vi "SVFA Get Spectrum Subset (1 Ch).vi"(0 "spectrum":cluster{"x0":dbl, "dx":dbl, "magnitude":dbl[]} {"magnitude" format="%.2f"; "dx" format="%.2f"; "x0" format="%.2f"}, 2 "range":cluster{"start":dbl, "stop":dbl}={"start"=-1.0, "stop"=-1.0} {"stop" format="%.2f"; "start" format="%.2f"}, 4 "spectrum info":T1={"channel name"="", "description"="", "x-axis units"=0, "spectral info"={"spectrum type"=enum."Power [Magnitude^2]", "linear/dB"=enum."linear", "window"=0, "window size"=0, "FFT size"=0}, "engineering units"=0, "custom label"="", "dB reference [EU]"=0.0, "peak units"=enum."rms", "weighting filter"=0, "spectral density?"=FALSE, "unit label"="", "spectrum skewed?"=FALSE, "complimentary spectrum units"=enum."none"} {"x-axis units" items=["Frequency-CB (Hz)"=0, "Frequency-CB (Hz)"=1, "Frequency-CPB (Hz)"=1248, "Frequency-Arbitrary (Hz)"=2357, "Quefrency (s)"=2, "Revolutions (rev)"=3, "Order"=4, "Speed (RPM)"=11, "Speed (rad/s)"=21, "Index"=65535]; "weighting filter" items=["Linear", "A-weighting", "B-weighting", "C-weighting", "ITU-R 468-4", "Dolby", "CCITT", "C-message", "Wb", "Wc", "Wd", "We", "Wf", "Wh", "Wj", "Wk", "Wm", "AES17 20 kHz lowpass", "AES17 40 kHz lowpass", "AES17 20 kHz highpass", "AES17 40 kHz highpass"]; "dB reference [EU]" format="%.2f"; "engineering units" items=["custom..."=0, "V"=1, "A"=21, "C"=30, "pC"=31, "s"=32, "-"=29, "Pa"=2, "N"=20, "g"=3, "m/s^2"=4, "m/s"=5, "m"=6, "mm/s"=12, "mm"=13, "micron/s"=14, "micron"=15, "in/s^2"=7, "in/s"=8, "in"=9, "mil/s"=10, "mil"=11, "rad/s^2"=16, "rad/s"=17, "rad"=18, "deg/s^2"=26, "deg/s"=27, "deg"=28, "RPM"=22, "cycle/s^2"=23, "Hz"=24, "cycle"=25, "strain"=19]; "spectral info"."window" items=["None "=0, "Hanning"=1, "Hamming"=2, "Blackman-Harris"=3, "Exact Blackman"=4, "Blackman"=5, "Flat Top"=6, "4 Term B-Harris "=7, "7 Term B-Harris"=8, "Low Sidelobe"=9, "Force - Exponential"=10, "Gaussian"=62]}, 5 "error in (no error)":errorcluster) -> (14 "spectrum subset":cluster{"x0":dbl, "dx":dbl, "magnitude":dbl[]} {"magnitude" format="%.2f"; "dx" format="%.2f"; "x0" format="%.2f"}, 15 "unit label":string, 16 "actual range":cluster{"start":dbl, "stop":dbl}={"start"=-1.0, "stop"=-1.0} {"stop" format="%.2f"; "start" format="%.2f"}, 17 "range label":string, 18 "dup spectrum info":T1={"channel name"="", "description"="", "x-axis units"=0, "spectral info"={"spectrum type"=enum."Power [Magnitude^2]", "linear/dB"=enum."linear", "window"=0, "window size"=0, "FFT size"=0}, "engineering units"=0, "custom label"="", "dB reference [EU]"=0.0, "peak units"=enum."rms", "weighting filter"=0, "spectral density?"=FALSE, "unit label"="", "spectrum skewed?"=FALSE, "complimentary spectrum units"=enum."none"} {"x-axis units" items=["Frequency-CB (Hz)"=0, "Frequency-CB (Hz)"=1, "Frequency-CPB (Hz)"=1248, "Frequency-Arbitrary (Hz)"=2357, "Quefrency (s)"=2, "Revolutions (rev)"=3, "Order"=4, "Speed (RPM)"=11, "Speed (rad/s)"=21, "Index"=65535]; "weighting filter" items=["Linear", "A-weighting", "B-weighting", "C-weighting", "ITU-R 468-4", "Dolby", "CCITT", "C-message", "Wb", "Wc", "Wd", "We", "Wf", "Wh", "Wj", "Wk", "Wm", "AES17 20 kHz lowpass", "AES17 40 kHz lowpass", "AES17 20 kHz highpass", "AES17 40 kHz highpass"]; "dB reference [EU]" format="%.2f"; "engineering units" items=["custom..."=0, "V"=1, "A"=21, "C"=30, "pC"=31, "s"=32, "-"=29, "Pa"=2, "N"=20, "g"=3, "m/s^2"=4, "m/s"=5, "m"=6, "mm/s"=12, "mm"=13, "micron/s"=14, "micron"=15, "in/s^2"=7, "in/s"=8, "in"=9, "mil/s"=10, "mil"=11, "rad/s^2"=16, "rad/s"=17, "rad"=18, "deg/s^2"=26, "deg/s"=27, "deg"=28, "RPM"=22, "cycle/s^2"=23, "Hz"=24, "cycle"=25, "strain"=19]; "spectral info"."window" items=["None "=0, "Hanning"=1, "Hamming"=2, "Blackman-Harris"=3, "Exact Blackman"=4, "Blackman"=5, "Flat Top"=6, "4 Term B-Harris "=7, "7 Term B-Harris"=8, "Low Sidelobe"=9, "Force - Exponential"=10, "Gaussian"=62]}, 19 "error out":errorcluster)   [LabVIEW 2017]
doc: "Extracts the subset of the spectrum specified by <B>range</B>. <B>x0</B> is updated to reflect the new start frequency, <B>dx</B> is the same as in the input spectrum, and the spectrum array is shortened so the last element corresponds with the stop value specified in the <B>range</B>. Use this VI for operations such as limiting subsequent spectrum operations to the region of interest or removing the part of the spectrum outside the alias-free bandwidth, as well as others. Wire data to the <B>spectrum</B> input to determine the polymorphic instance to use or manually select the instance."
uses:
  <vilib>/addons/_NISVFA/_Shared subVIs/Controls/svc_Spectrum Info.ctl
  <vilib>/addons/_NISVFA/_Shared subVIs/Controls/svc_X-Axis Units.ctl
  <vilib>/addons/_NISVFA/_Shared subVIs/Controls/svc_Spectrum Type.ctl
  <vilib>/addons/_NISVFA/_Shared subVIs/Controls/svc_Engineering Units Text Ring.ctl
  <vilib>/addons/_NISVFA/_Shared subVIs/Controls/svc_Weighting Filter Text Ring.ctl
  <vilib>/addons/_NISVFA/_Shared subVIs/Controls/svc_Complimentary Spectrum Units.ctl
  <vilib>/addons/_NISVFA/_Shared subVIs/Common/svc_Get Weighting Enum and Labels.vi
  <vilib>/addons/_NISVFA/_Shared subVIs/Common/svc_Unit Label Lexical Class.vi
  <vilib>/addons/_NISVFA/_Shared subVIs/Common/svc_Engineering Units to Unit Label.vi
  <vilib>/addons/_NISVFA/_Shared subVIs/Common/svc_Format Value (DBL).vi
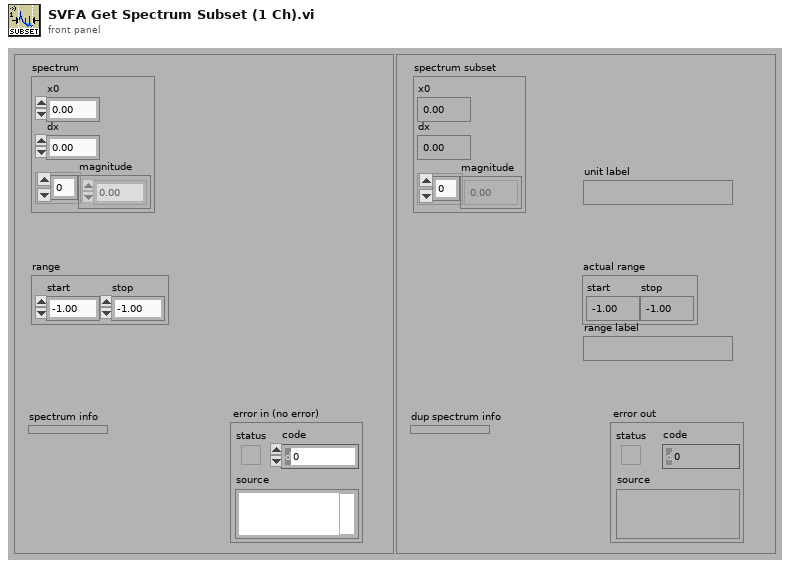
[diagram p1: front panel]
types:
  T1 = typedef "svc_Spectrum Info.ctl" = cluster{"channel name":string, "description":string, "x-axis units":T2, "spectral info":cluster{"spectrum type":T3, "linear/dB":enum16{"linear", "dB"}, "window":u16, "window size":i32, "FFT size":i32}, "engineering units":T4, "custom label":string, "dB reference [EU]":dbl, "peak units":enum16{"rms", "peak", "peak-peak"}, "weighting filter":T5, "spectral density?":bool, "unit label":string, "spectrum skewed?":bool, "complimentary spectrum units":T6}
  T2 = typedef "svc_X-Axis Units.ctl" = u16
  T3 = typedef "svc_Spectrum Type.ctl" = enum16{"FFT Spectrum [complex]", "Amplitude [Magnitude]", "Power [Magnitude^2]", "Cross Spectrum [complex]", "Frequency Response [Complex]"}
  T4 = typedef "svc_Engineering Units Text Ring.ctl" = u16
  T5 = typedef "svc_Weighting Filter Text Ring.ctl" = u16
  T6 = typedef "svc_Complimentary Spectrum Units.ctl" = enum16{"none", "radians", "degrees", "cycles", "imaginary"}
  T7 = cluster{"start frequency":dbl, "stop frequency":dbl}
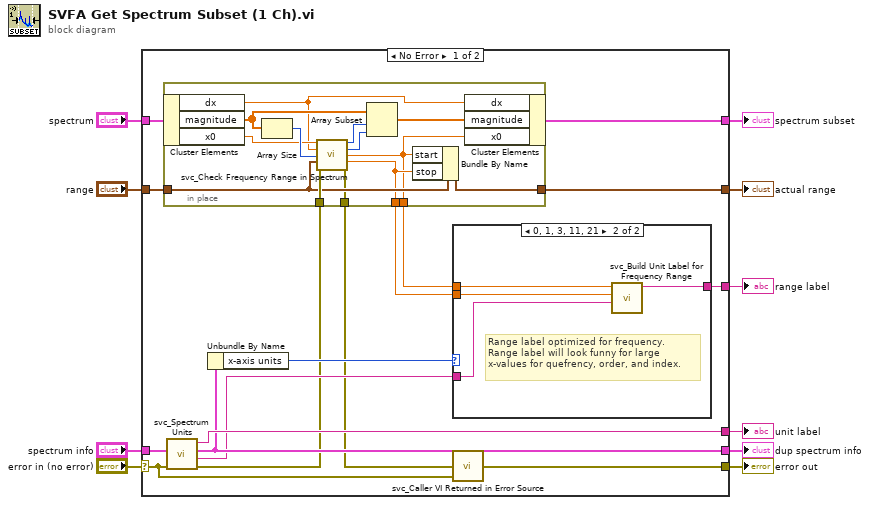
[diagram p0: block diagram]
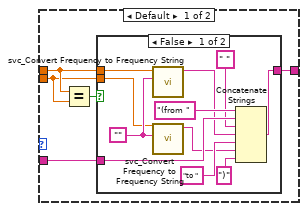
[diagram p2: hidden frame]
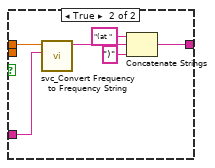
[diagram p3: hidden frame]
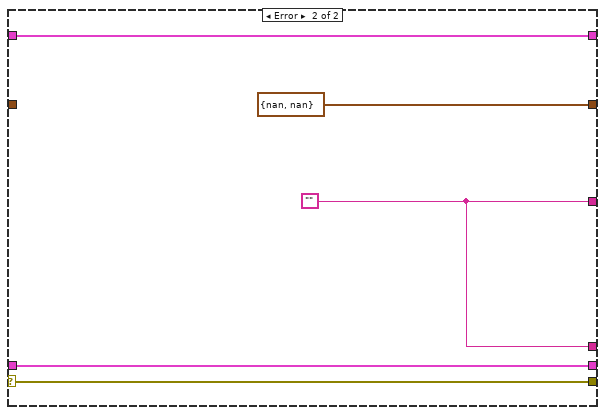
[diagram p4: hidden frame]
diagram:
  n1 = case shown="No Error" "error in (no error)" {
    selector: "error in (no error)" -> [w13 w69]
    tunnel: [w11 w70] -> w10
    tunnel: "range" -> [w17 _]
    tunnel: "spectrum" -> [w12 w70]
    tunnel: [w25 w66] -> w6
    tunnel: [w23 w68] -> w3
    tunnel: "spectrum info" -> [w19 w68]
    tunnel: [w24 T7 {"start frequency"=nan, "stop frequency"=nan} ("frequency range")] -> w2
    tunnel: [w14 w69] -> w9
    tunnel: [w26 w66] -> w1
    frame No Error {
      n2 = call <vilib>:"svc_Spectrum Units.vi"("error in (no error)"=w13, "spectrum info in"=w19) -> ("error out"=w20:errorcluster, "x-axis unit label"=w21:string, "spectrum info out"=w23:T1, "unit label"=w26:string)  [unwired: 2 in]
      n3 = in-place {
        in-place-border: [w36] -> w24
        in-place-border: w20 -> [w35]
        in-place-border: [w28] -> w18
        in-place-border: w17 -> [w34]
        in-place-border: [w33] -> w16
        in-place-border: [w32] -> w15
        n4 = in-place-cluster #1(w12) -> ("dx"=w27:dbl, "magnitude"=w31:dbl[], "x0"=w30:dbl)
        n5 = Array Size(array=w31) -> (size(s)=w37:i32)
        n6 = call <vilib>:"svc_Check Frequency Range in Spectrum.vi"("f0"=w30, "df"=w27, "spectrum length"=w37, "frequency range"=w34, "error in (no error)"=w35) -> ("start index"=w38:i32, "band length"=w39:i32, "f0"=w28:dbl, "fmax"=w33:dbl, "error out"=w32:errorcluster)  [unwired: 6 in]
        n7 = Array Subset(array=w31, index=w38, length=w39) -> (w29:dbl[])
        n8 = Bundle By Name(cluster=w34, "start"=w28, "stop"=w33) -> (w36:cluster{"start":dbl, "stop":dbl})
        n9 = in-place-cluster #1("dx"=w27, "magnitude"=w29, "x0"=w28) -> (w11:cluster{"x0":dbl, "dx":dbl, "magnitude":dbl[]})
      }
      n10 = Unbundle By Name(w23) -> ("x-axis units"=w22:T2)
      n11 = case shown="0, 1, 3, 11, 21" w22 {
        tunnel: w16 -> [w41 w65]
        tunnel: w18 -> [w42 w64]
        tunnel: [w43 w63] -> w25
        tunnel: w21 -> [w44 w62]
        frame Default {
          n12 = Equal?(x=w42, y=w41) -> (x = y?=w40:bool)
          n13 = case shown="False" w40 {
            tunnel: w44 -> [w53 w60]
            tunnel: [w49 w56] -> w43
            tunnel: w42 -> [w48 w61]
            tunnel: w41 -> [w47 _]
            frame False {
              w55 = "" ("Empty String Constant")
              n14 = call <vilib>:"svc_Convert Frequency to Frequency String.vi"("x-axis unit label"=w55, "frequency [Hz]"=w48) -> ("frequency string"=w52:string)  [unwired: 9 in]
              n15 = call <vilib>:"svc_Convert Frequency to Frequency String.vi"("x-axis unit label"=w55, "frequency [Hz]"=w47) -> ("frequency string"=w46:string)  [unwired: 9 in]
              n16 = Concatenate Strings("(from ", w53, " ", w52, "to ", w46, ")") -> (w49:string)
            }
            frame True {
              n17 = call <vilib>:"svc_Convert Frequency to Frequency String.vi"("x-axis unit label"=w60, "frequency [Hz]"=w61) -> ("frequency string"=w58:string)  [unwired: 9 in]
              n18 = Concatenate Strings("(at " ("string"), w58, ")" ("string")) -> (w56:string)
            }
          }
        }
        frame 0, 1, 3, 11, 21 {
          # "Range label optimized for frequency.\nRange label will look funny for large \nx-values for quefrency, order, and index."
          n19 = call <vilib>:"svc_Build Unit Label for Frequency Range.vi"("x-axis unit label"=w62, "fmax"=w65, "f0"=w64) -> ("frequency range string"=w63:string)  [unwired: 8 in]
        }
      }
      n20 = call <vilib>:"svc_Caller VI Returned in Error Source.vi"("warning input to caller"=w13, "error in (no error)"=w15) -> ("error out"=w14:errorcluster)  [unwired: 3 in]
    }
    frame Error {
      w66 = "" ("frequency range string")
    }
  }
  "error out" <- w9
  "spectrum subset" <- w10
  "dup spectrum info" <- w3
  "range label" <- w6
  "actual range" <- w2
  "unit label" <- w1
